vi "Replace BD Decoration Text by Content.vi"(8 "error in":errorcluster, 9 "New Content":string, 10 "Old (partial) Content":string, 11 "VI  Ref":refnum<vi>) -> (0 "error out":errorcluster, 1 "Old Content":string, 2 "VI Modified & Saved?":bool, 3 "VI  Ref (dup)":refnum<vi>)   [LabVIEW 2021, in "Utilities.lvlib"]
doc: "Finds decorations in the diagram and looks for those containing the <B>Old (partial) Content</B> string.\n\nIf found, the decoration's content is replaced by <B>New Content</B>.\n\nNote that the comparison casts both input and content to lowercase characters."
uses:
  Utilities.lvlib
panel:
  # "see the AlliGator License on the block diagram (Ctrl+E or Window:Show Block Diagram)"
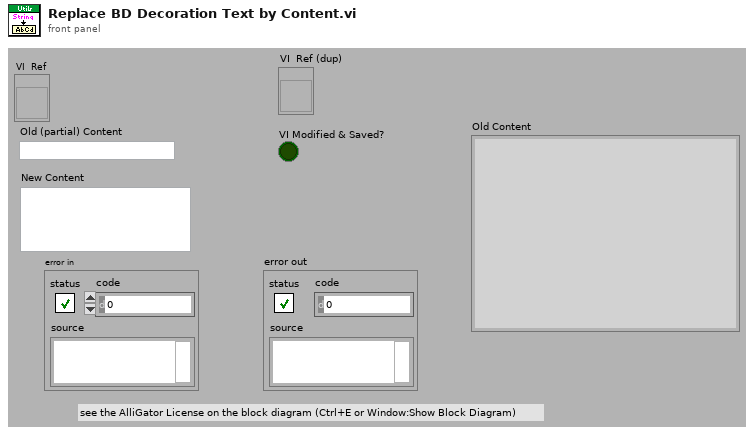
[diagram p1: front panel]
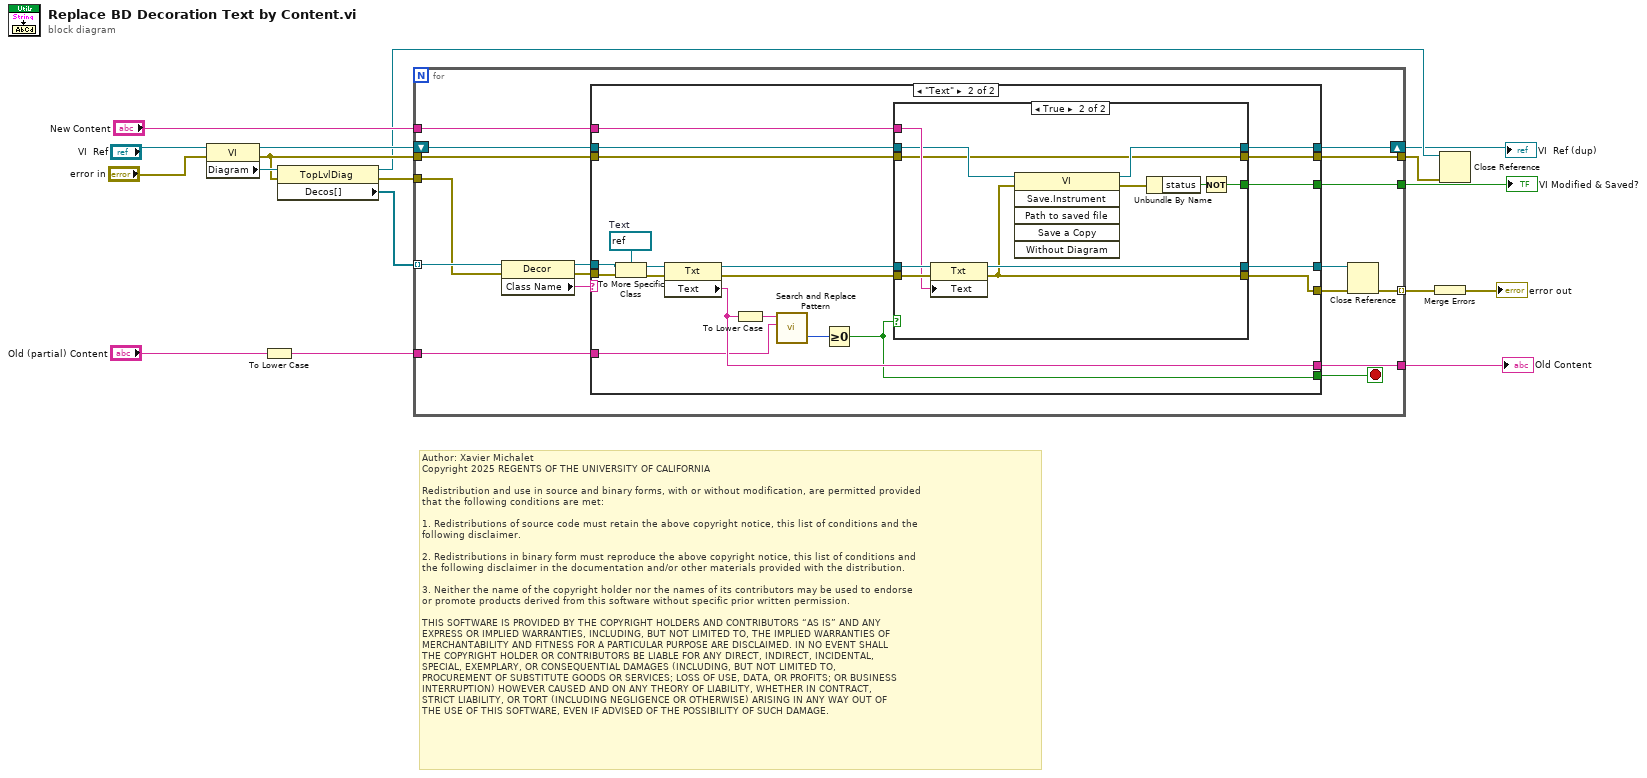
[diagram p0: block diagram]
diagram:
  # "Author: Xavier Michalet\nCopyright 2025 REGENTS OF THE UNIVERSITY OF CALIFORNIA\n\nRedistribution and use in source and binary forms, with or without modification, are permitted provided\nthat the following conditions are met:\n\n1. Redistributions of source code must retain the above copyright notice, this list of conditions and the\nfollowing disclaimer.\n\n2. Redistributions in binary form must reproduce the above copyright notice, this list of conditions and\nthe following disclaimer in the documentation and/or other materials provided with the distribution.\n\n3. Neither the name of the copyright holder nor the names of its contributors may be used to endorse \nor promote products derived from this software without specific prior written permission.\n\nTHIS SOFTWARE IS PROVIDED BY THE COPYRIGHT HOLDERS AND CONTRIBUTORS “AS IS” AND ANY \nEXPRESS OR IMPLIED WARRANTIES, INCLUDING, BUT NOT LIMITED TO, THE IMPLIED WARRANTIES OF\nMERCHANTABILITY AND FITNESS FOR A PARTICULAR PURPOSE ARE DISCLAIMED. IN NO EVENT SHALL\nTHE COPYRIGHT HOLDER OR CONTRIBUTORS BE LIABLE FOR ANY DIRECT, INDIRECT, INCIDENTAL, \nSPECIAL, EXEMPLARY, OR CONSEQUENTIAL DAMAGES (INCLUDING, BUT NOT LIMITED TO, \nPROCUREMENT OF SUBSTITUTE GOODS OR SERVICES; LOSS OF USE, DATA, OR PROFITS; OR BUSINESS\nINTERRUPTION) HOWEVER CAUSED AND ON ANY THEORY OF LIABILITY, WHETHER IN CONTRACT, \nSTRICT LIABILITY, OR TORT (INCLUDING NEGLIGENCE OR OTHERWISE) ARISING IN ANY WAY OUT OF\nTHE USE OF THIS SOFTWARE, EVEN IF ADVISED OF THE POSSIBILITY OF SUCH DAMAGE."
  n1 = property class="VI"(reference="VI  Ref", error in="error in") -> (reference out=w8:refnum<vi>, error out=w7:errorcluster, "Diagram"=w16:refnum<vi>)
  n2 = To Lower Case(string="Old (partial) Content") -> (all lower case string=w1:string)
  n3 = property class="TopLvlDiag"(reference=w16, error in=w7) -> (reference out=w4:refnum<vi>, error out=w15:errorcluster, "Decos[]"=w17:refnum<vi>[])
  n4 = for {
    tunnel: w1 -> [w32]
    tunnel: w17 -> [w28] mode=indexing
    tunnel: w15 -> [w19]
    tunnel: [w29] -> w14 mode=indexing
    tunnel: [w25] -> w10
    tunnel: "New Content" -> [w24]
    tunnel: w7 -> [w22]
    tunnel: [w21] -> w5
    tunnel: [w18] -> w2
    shift-right: [w20] -> w3
    shift-left: w8 -> [w23]
    stop <- w27 stop-if-true
    n5 = property class="Decor"(reference=w28, error in=w19) -> (reference out=w34:refnum<vi>, error out=w33:errorcluster, "Class Name"=w26:string)
    n6 = case shown="\"Text\"" w26 {
      tunnel: w34 -> [w38 w57]
      tunnel: w33 -> [w37 w58]
      tunnel: [w37 w50] -> w30
      tunnel: w32 -> [_ w41]
      tunnel: [w38 w51] -> w31
      tunnel: [_ w39] -> w27
      tunnel: [_ w43] -> w25
      tunnel: w24 -> [_ w49]
      tunnel: w23 -> [w36 w48]
      tunnel: w22 -> [w35 w47]
      tunnel: [_ w46] -> w21
      tunnel: [w36 w45] -> w20
      tunnel: [w35 w44] -> w18
      frame "", Default {
      }
      frame "Text" {
        w56 = refnum<vi> refnum  # Text
        n7 = To More Specific Class(target class=w56, reference=w57, error in=w58) -> (specific class reference=w55:refnum<vi>, error out=w54:errorcluster)
        n8 = property class="Txt"(reference=w55, error in=w54) -> (reference out=w53:refnum<vi>, error out=w52:errorcluster, "Text"=w43:string)
        n9 = To Lower Case(string=w43) -> (all lower case string=w42:string)
        n10 = call <vilib>:"Search and Replace Pattern.vi"("string"=w42, "regular expression (\"\")"=w41) -> ("offset past match"=w40:i32)  [unwired: 3 in, 1 out]
        n11 = Greater Or Equal To 0?(x=w40) -> (x >= 0?=w39:bool)
        n12 = case shown="True" w39 {
          tunnel: w53 -> [w62 w73]
          tunnel: w52 -> [w61 w72]
          tunnel: [w62 w68] -> w51
          tunnel: [w61 w67] -> w50
          tunnel: w49 -> [_ w71]
          tunnel: w48 -> [w60 w70]
          tunnel: [w60 w69] -> w45
          tunnel: w47 -> [w59 w63]
          tunnel: [_ w64] -> w46
          tunnel: [w59 w63] -> w44
          frame False {
          }
          frame True {
            n13 = property class="Txt"(reference=w73, error in=w72, "Text"=w71) -> (reference out=w68:refnum<vi>, error out=w67:errorcluster)
            n14 = invoke class="VI" method="Save.Instrument"(reference=w70, error in=w67) -> (reference out=w69:refnum<vi>, error out=w66:errorcluster)  [unwired: 4 in, 4 out]
            n15 = Unbundle By Name(w66) -> ("status"=w65:bool)
            n16 = Not(x=w65) -> (.not. x?=w64:bool)
          }
        }
      }
    }
    n17 = Close Reference(reference=w31, error in (no error)=w30) -> (error out=w29:errorcluster)
  }
  "Old Content" <- w10
  "VI Modified & Saved?" <- w5
  "VI  Ref (dup)" <- w3
  n18 = Merge Errors(w14) -> (→"error out":errorcluster)
  n19 = Close Reference(reference=w4, error in (no error)=w2) -> ()  [unwired: 1 out]
